vi "XY to Velocity.vi"(2 "Expo":dbl(slide) scale=0.0..100.0, 3 "Nunchuk Analog Stick In":cluster{"X":dbl, "Y":dbl}) -> (0 "X and Y":cluster{"X":dbl, "Y":dbl}, 1 "Nunchuk Analog Stick":cluster{dbl, dbl}[](graph))   [LabVIEW 2011]
panel:
  out "X":dbl
  out "Y":dbl
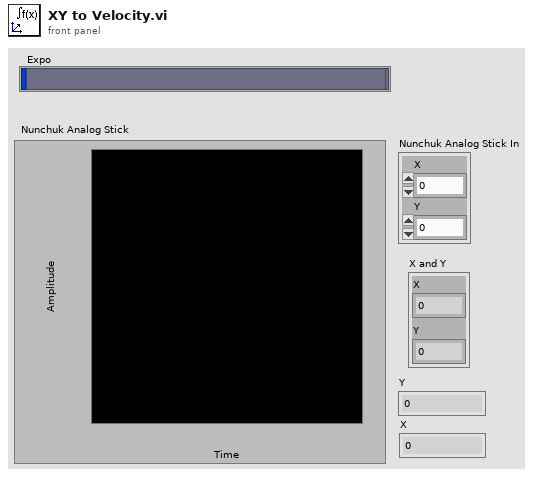
[diagram p1: front panel]
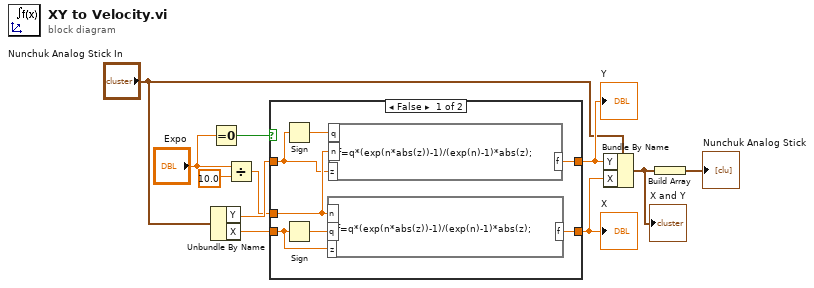
[diagram p0: block diagram]
diagram:
  n1 = Equal To 0?(x="Expo") -> (x = 0?=w7:bool)
  n2 = Unbundle By Name("Nunchuk Analog Stick In") -> ("Y"=w11:dbl, "X"=w3:dbl)
  n3 = Divide(x="Expo", y=10.0) -> (x/y=w5:dbl)
  n4 = case shown="False" w7 {
    tunnel: w11 -> [w12 w20]
    tunnel: w3 -> [w15 w19]
    tunnel: [w18 w20] -> w9
    tunnel: [w17 w19] -> w8
    tunnel: w5 -> [w16 _]
    frame False {
      n5 = Sign(1:w12) -> (0:w13:dbl)
      n6 = Sign(1:w15) -> (0:w14:dbl)
      n7 = formula code="f=q*(exp(n*abs(z))-1)/(exp(n)-1)*abs(z);"("n"=w16, "z"=w15, "q"=w14) -> ("f"=w17:dbl)
      n8 = formula code="f=q*(exp(n*abs(z))-1)/(exp(n)-1)*abs(z);"("n"=w16, "z"=w12, "q"=w13) -> ("f"=w18:dbl)
    }
    frame True {
    }
  }
  "Y" <- w9
  "X" <- w8
  n9 = Bundle By Name(cluster="Nunchuk Analog Stick In", "Y"=w9, "X"=w8) -> (w2:cluster{"X":dbl, "Y":dbl})
  "X and Y" <- w2
  n10 = Build Array(w2) -> (→"Nunchuk Analog Stick":cluster{"X":dbl, "Y":dbl}[])
